vi "StatTable_Popup.vi"() -> ()   [LabVIEW 2010]
uses:
  <vilib>/Utility/miscctls.llb/LVRowAndColumnTypeDef.ctl
panel:
  in  "z_#":i32=8 caption="# columns"
  in  "z_Cell Width":u32
  in  "Resize":bool
  in  "Close":bool
  in  "Table":string[][](table)=[["test1", "test2", "test3", "test4", "", "", "", ""], ["0", "0", "0", "0", "0", "0", "0", "0"], ["0", "0", "0", "0", "0", "0", "0", "0"], ["0", "0", "0", "0", "0", "0", "0", "0"], ["0", "0", "0", "0", "0", "0", "0", "0"], ["0", "0", "0", "0", "0", "0", "0", "0"], ["0", "0", "0", "0", "0", "0", "0", "0"], ["0", "0", "0", "0", "0", "0", "0", "0"], ["0", "0", "0", "0", "0", "0", "0", "0"], ["0", "0", "0", "0", "0", "0", "0", "0"], ["0", "0", "0", "0", "0", "0", "0", "0"]]
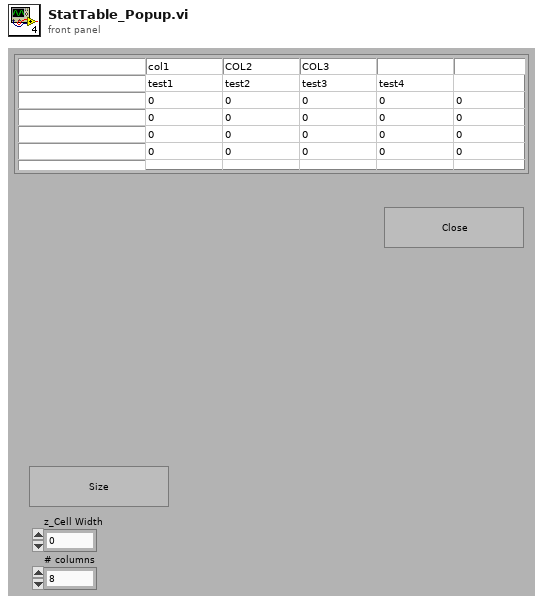
[diagram p1: front panel]
types:
  T1 = typedef "LVRowAndColumnTypeDef.ctl" = cluster{"Row":i32, "Column":i32}
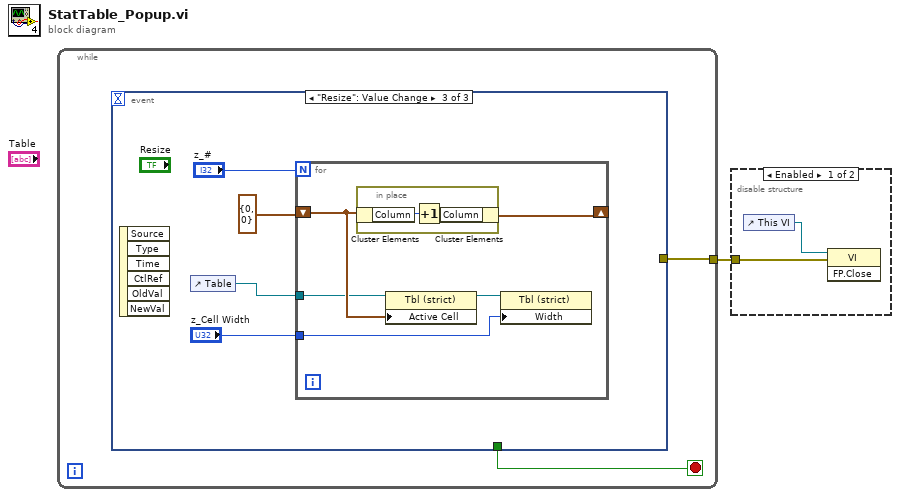
[diagram p0: block diagram]
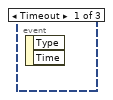
[diagram p3: hidden frame]
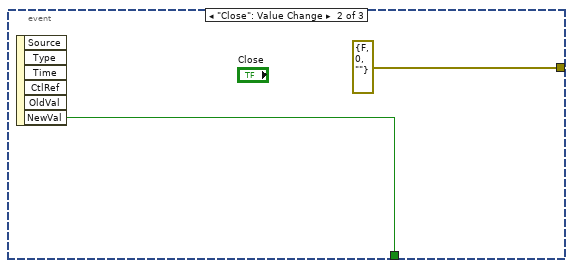
[diagram p4: hidden frame]
diagram:
  n1 = while {
    tunnel: [w2] -> w1
    stop <- w3 stop-if-true
    n2 = event shown="[2] \"Resize\": Value Change" {
      selector: _ -> [_ _ _]
      dyn-events: _ -> [_ _ _]
      timeout: _ -> [_ _ _]
      tunnel: [_ w5 _] -> w3
      tunnel: [_ errorcluster {"status"=FALSE, "code"=0, "source"=""} ("error in (no error)") _] -> w2
      event Timeout {
        n3 = event-data() -> ()  [unwired: 3 out]
      }
      event "Close": Value Change {
        n4 = event-data() -> ("NewVal"=w5:bool)  [unwired: 6 out]
      }
      event "Resize": Value Change {
        n5 = event-data() -> ()  [unwired: 7 out]
        n6 = control-ref of="Table"() -> (w9:refnum<vi>)
        n7 = for {
          N: "z_#" -> [_]
          tunnel: "z_Cell Width" -> [w13]
          shift-right: [w14] -> _
          shift-left: T1 {"Row"=0, "Column"=0} ("Active Cell:Active Cell") -> [w12]
          tunnel: w9 -> [w11]
          n8 = in-place "In Place Element Structure" {
            n9 = in-place-cluster #1(w12) -> ("Column"=w15:i32)
            n10 = Increment(x=w15) -> (x+1=w16:i32)
            n11 = in-place-cluster #1("Column"=w16) -> (w14:T1)
          }
          n12 = property on="Property Node" class="Tbl (strict)"(reference=w11, "Active Cell"=w12) -> (reference out=w10:refnum<vi>)  [unwired: 1 in, 1 out]
          n13 = property on="Property Node" class="Tbl (strict)"(reference=w10, "Width"=w13) -> ()  [unwired: 1 in, 2 out]
        }
      }
    }
  }
  n14 = disable-structure shown="Enabled" {
    disable-tunnel: w1 -> [w17 _]
    frame Enabled {
      n15 = control-ref of="This VI"() -> (w18:refnum<vi>)
      n16 = invoke class="VI" method="FP.Close"(reference=w18, error in=w17) -> ()  [unwired: 1 in, 3 out]
    }
    frame Disabled {
    }
  }
